vi "__SET_PM_1ch_E4419A.VI"(5 "aveg":i32=1, 6 "frq(GHz)":dbl=12.0, 7 "GPIB":string="13") -> ()   [LabVIEW 2017]
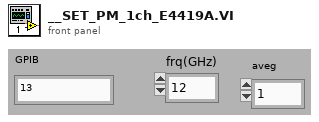
[diagram p1: front panel]
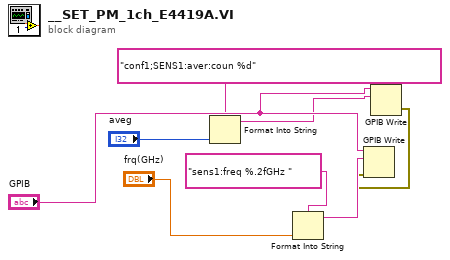
[diagram p0: block diagram]
diagram:
  n1 = Format Into String(format string="conf1;SENS1:aver:coun %d", "aveg") -> (resulting string=w5:string)  [unwired: 2 in, 1 out]
  n2 = Format Into String(format string="sens1:freq %.2fGHz ", "frq(GHz)") -> (resulting string=w2:string)  [unwired: 2 in, 1 out]
  n3 = GPIB Write(0:"GPIB", 1:w5) -> (6:w1:errorcluster)  [unwired: 3 in, 1 out]
  n4 = GPIB Write(0:"GPIB", 1:w2, 3:w1) -> ()  [unwired: 2 in, 2 out]
